vi "SensorSimulationTool.vi"() -> ()   [LabVIEW 2023]
panel:
  in  "ClientUI":enum32{"Page 2"}(tab)
  in  "Bypass1":bool
  in  "Bypass2":bool
  in  "Bypass3":bool
  in  "Bypass4":bool
  in  "Bypass5":bool
  in  "Bypass6":bool
  in  "Tamper1":bool
  in  "Tamper2":bool
  in  "Tamper3":bool
  in  "Tamper4":bool
  in  "Tamper5":bool
  in  "Tamper6":bool
  in  "Alarm1":bool
  in  "Alarm2":bool
  in  "Alarm4":bool
  in  "Alarm5":bool
  in  "Alarm6":bool
  in  "stop":bool
  in  "Alarm3":bool
  # "Zone Sensor Simulation Panel"
  # "1"
  # "2"
  # "3"
  # "4"
  # "5"
  # "6"
  # "Zone"
  # "Alarm Switches"
  # "Bypass Switches"
  # "Tamper Switches"
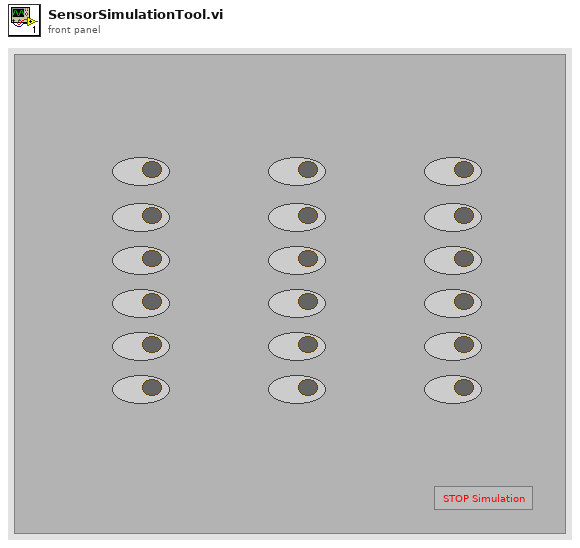
[diagram p1: front panel]
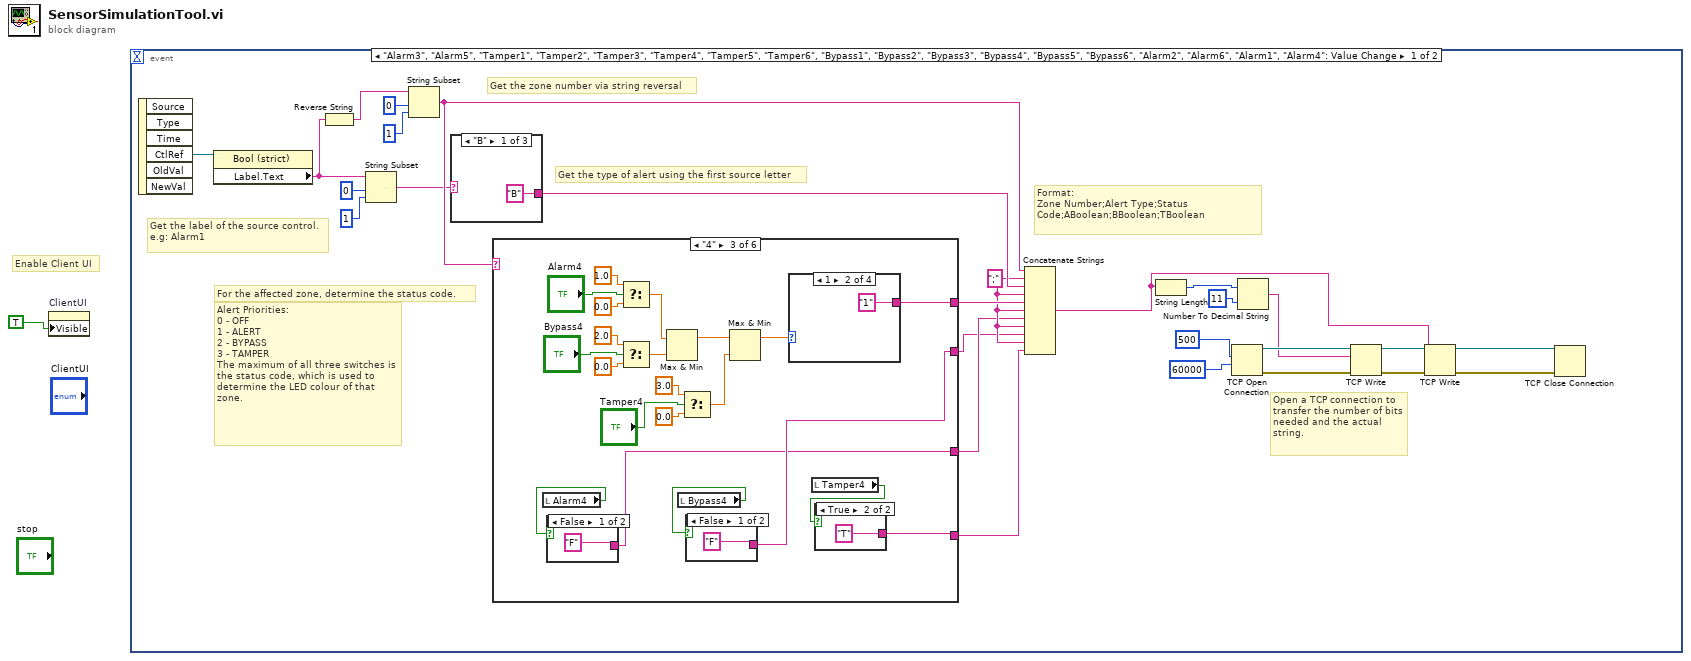
[diagram p0: block diagram]
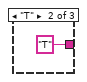
[diagram p2: hidden frame]
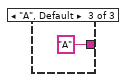
[diagram p3: hidden frame]
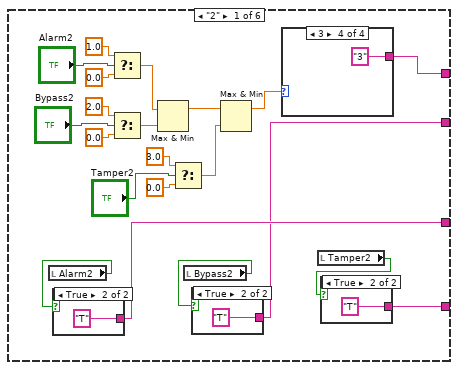
[diagram p4: hidden frame]
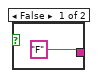
[diagram p5: hidden frame]
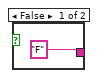
[diagram p6: hidden frame]
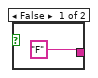
[diagram p7: hidden frame]
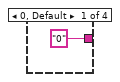
[diagram p8: hidden frame]
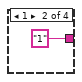
[diagram p9: hidden frame]
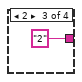
[diagram p10: hidden frame]
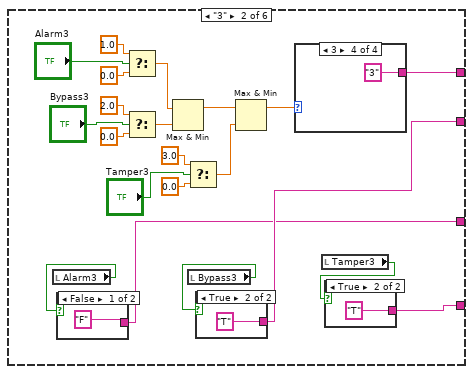
[diagram p11: hidden frame]
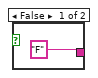
[diagram p12: hidden frame]
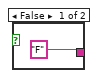
[diagram p13: hidden frame]
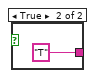
[diagram p14: hidden frame]
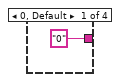
[diagram p15: hidden frame]
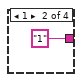
[diagram p16: hidden frame]
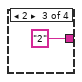
[diagram p17: hidden frame]
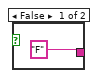
[diagram p18: hidden frame]
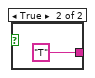
[diagram p19: hidden frame]
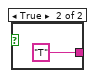
[diagram p20: hidden frame]
diagram:
  # "Enable Client UI"
  n1 = property on="ClientUI" class="TabCtl (strict)"("Visible"=TRUE) -> ()  [unwired: 2 in, 2 out]
  n2 = event shown="[0] \"Alarm3\", \"Alarm5\", \"Tamper1\", \"Tamper2\", \"Tamper3\", \"Tamper4\", \"Tamper5\", \"Tamper6\", \"Bypass1\", \"Bypass2\", \"Bypass3\", \"Bypass4\", \"Bypass5\", \"Bypass6\", \"Alarm2\", \"Alarm6\", \"Alarm1\", \"Alarm4\": Value Change" {
    selector: _ -> [_ _]
    dyn-events: _ -> [_ _]
    timeout: _ -> [_ _]
    event "Alarm3", "Alarm5", "Tamper1", "Tamper2", "Tamper3", "Tamper4", "Tamper5", "Tamper6", "Bypass1", "Bypass2", "Bypass3", "Bypass4", "Bypass5", "Bypass6", "Alarm2", "Alarm6", "Alarm1", "Alarm4": Value Change {
      w8 = ";" ("string")
      # "Open a TCP connection to transfer the number of bits needed and the actual string."
      # "Alert Priorities:\n0 - OFF\n1 - ALERT\n2 - BYPASS\n3 - TAMPER\nThe maximum of all three switches is the status code, which is used to determine the LED colour of that zone."
      # "For the affected zone, determine the status code."
      # "Get the type of alert using the first source letter"
      # "Get the zone number via string reversal"
      # "Get the label of the source control. e.g: Alarm1"
      # "Format:\nZone Number;Alert Type;Status Code;ABoolean;BBoolean;TBoolean"
      n3 = event-data() -> ("CtlRef"=w22:refnum<vi>)  [unwired: 1 in, 5 out]
      n4 = property class="Bool (strict)"(reference=w22) -> ("Label.Text"=w15:string)  [unwired: 1 in, 2 out]
      n5 = Reverse String(1:w15) -> (0:w19:string)
      n6 = String Subset(string=w15, offset (0)=0, length (rest)=1 ("length (rest)")) -> (substring=w12:string)
      n7 = String Subset(string=w19, offset (0)=0, length (rest)=1 ("length (rest)")) -> (substring=w16:string)
      n8 = case shown="\"B\"" w12 {
        tunnel: ["B" ("string") "T" ("string") "A" ("string")] -> w10
        frame "B" {
        }
        frame "T" {
        }
        frame "A", Default {
        }
      }
      n9 = case shown="\"4\"" w16 {
        tunnel: [w41 w72 w100 w134 w162 w193] -> w11
        tunnel: [w33 w63 w94 w125 w156 w187] -> w7
        tunnel: [w32 w64 w95 w126 w157 w188] -> w6
        tunnel: [w37 w68 w99 w130 w161 w192] -> w5
        frame "2" {
          n10 = local read "Alarm2"() -> (w36:bool)
          n11 = case shown="True" w36 {
            tunnel: ["F" "T"] -> w33
            frame False {
            }
            frame True {
            }
          }
          n12 = Select(t=1.0, s="Alarm2", f=0.0) -> (s? t:f=w46:dbl)
          n13 = Select(t=2.0, s="Bypass2", f=0.0) -> (s? t:f=w45:dbl)
          n14 = Max & Min(x=w46, y=w45) -> (max(x,y)=w44:dbl)  [unwired: 1 out]
          n15 = Select(t=3.0, s="Tamper2", f=0.0) -> (s? t:f=w43:dbl)
          n16 = local read "Bypass2"() -> (w35:bool)
          n17 = case shown="True" w35 {
            tunnel: ["F" "T"] -> w32
            frame False {
            }
            frame True {
            }
          }
          n18 = Max & Min(x=w44, y=w43) -> (max(x,y)=w42:dbl)  [unwired: 1 out]
          n19 = case shown="3" w42 {
            tunnel: ["0" "1" "2" "3"] -> w41
            frame 0, Default {
            }
            frame 1 {
            }
            frame 2 {
            }
            frame 3 {
            }
          }
          n20 = local read "Tamper2"() -> (w34:bool)
          n21 = case shown="True" w34 {
            tunnel: ["F" "T"] -> w37
            frame False {
            }
            frame True {
            }
          }
        }
        frame "3" {
          n22 = local read "Alarm3"() -> (w67:bool)
          n23 = case shown="False" w67 {
            tunnel: ["F" "T"] -> w63
            frame False {
            }
            frame True {
            }
          }
          n24 = Select(t=1.0, s="Alarm3", f=0.0) -> (s? t:f=w77:dbl)
          n25 = Select(t=2.0, s="Bypass3", f=0.0) -> (s? t:f=w76:dbl)
          n26 = Max & Min(x=w77, y=w76) -> (max(x,y)=w75:dbl)  [unwired: 1 out]
          n27 = Select(t=3.0, s="Tamper3", f=0.0) -> (s? t:f=w74:dbl)
          n28 = local read "Bypass3"() -> (w66:bool)
          n29 = case shown="True" w66 {
            tunnel: ["F" "T"] -> w64
            frame False {
            }
            frame True {
            }
          }
          n30 = Max & Min(x=w75, y=w74) -> (max(x,y)=w73:dbl)  [unwired: 1 out]
          n31 = case shown="3" w73 {
            tunnel: ["0" "1" "2" "3"] -> w72
            frame 0, Default {
            }
            frame 1 {
            }
            frame 2 {
            }
            frame 3 {
            }
          }
          n32 = local read "Tamper3"() -> (w65:bool)
          n33 = case shown="True" w65 {
            tunnel: ["F" "T"] -> w68
            frame False {
            }
            frame True {
            }
          }
        }
        frame "4" {
          n34 = local read "Alarm4"() -> (w98:bool)
          n35 = case shown="False" w98 {
            tunnel: ["F" "T"] -> w94
            frame False {
            }
            frame True {
            }
          }
          n36 = Select(t=1.0, s="Alarm4", f=0.0) -> (s? t:f=w108:dbl)
          n37 = Select(t=2.0, s="Bypass4", f=0.0) -> (s? t:f=w107:dbl)
          n38 = Max & Min(x=w108, y=w107) -> (max(x,y)=w106:dbl)  [unwired: 1 out]
          n39 = local read "Bypass4"() -> (w97:bool)
          n40 = Select(t=3.0, s="Tamper4", f=0.0) -> (s? t:f=w105:dbl)
          n41 = case shown="False" w97 {
            tunnel: ["F" "T"] -> w95
            frame False {
            }
            frame True {
            }
          }
          n42 = Max & Min(x=w106, y=w105) -> (max(x,y)=w104:dbl)  [unwired: 1 out]
          n43 = case shown="1" w104 {
            tunnel: ["0" "1" "2" "3"] -> w100
            frame 0, Default {
            }
            frame 1 {
            }
            frame 2 {
            }
            frame 3 {
            }
          }
          n44 = local read "Tamper4"() -> (w96:bool)
          n45 = case shown="True" w96 {
            tunnel: ["F" "T"] -> w99
            frame False {
            }
            frame True {
            }
          }
        }
        frame "5" {
          n46 = local read "Alarm5"() -> (w129:bool)
          n47 = case shown="True" w129 {
            tunnel: ["F" "T"] -> w125
            frame False {
            }
            frame True {
            }
          }
          n48 = Select(t=1.0, s="Alarm5", f=0.0) -> (s? t:f=w139:dbl)
          n49 = Select(t=2.0, s="Bypass5", f=0.0) -> (s? t:f=w138:dbl)
          n50 = Max & Min(x=w139, y=w138) -> (max(x,y)=w137:dbl)  [unwired: 1 out]
          n51 = local read "Bypass5"() -> (w128:bool)
          n52 = case shown="False" w128 {
            tunnel: ["F" "T"] -> w126
            frame False {
            }
            frame True {
            }
          }
          n53 = Select(t=3.0, s="Tamper5", f=0.0) -> (s? t:f=w136:dbl)
          n54 = Max & Min(x=w137, y=w136) -> (max(x,y)=w135:dbl)  [unwired: 1 out]
          n55 = case shown="1" w135 {
            tunnel: ["0" "1" "2" "3"] -> w134
            frame 0, Default {
            }
            frame 1 {
            }
            frame 2 {
            }
            frame 3 {
            }
          }
          n56 = local read "Tamper5"() -> (w127:bool)
          n57 = case shown="False" w127 {
            tunnel: ["F" "T"] -> w130
            frame False {
            }
            frame True {
            }
          }
        }
        frame "6" {
          n58 = local read "Alarm6"() -> (w160:bool)
          n59 = case shown="False" w160 {
            tunnel: ["F" "T"] -> w156
            frame False {
            }
            frame True {
            }
          }
          n60 = Select(t=1.0, s="Alarm6", f=0.0) -> (s? t:f=w172:dbl)
          n61 = Select(t=2.0, s="Bypass6", f=0.0) -> (s? t:f=w173:dbl)
          n62 = local read "Bypass6"() -> (w159:bool)
          n63 = Max & Min(x=w172, y=w173) -> (max(x,y)=w174:dbl)  [unwired: 1 out]
          n64 = case shown="True" w159 {
            tunnel: ["F" "T"] -> w157
            frame False {
            }
            frame True {
            }
          }
          n65 = Select(t=3.0, s="Tamper6", f=0.0) -> (s? t:f=w175:dbl)
          n66 = Max & Min(x=w174, y=w175) -> (max(x,y)=w176:dbl)  [unwired: 1 out]
          n67 = case shown="3" w176 {
            tunnel: ["0" "1" "2" "3"] -> w162
            frame 0, Default {
            }
            frame 1 {
            }
            frame 2 {
            }
            frame 3 {
            }
          }
          n68 = local read "Tamper6"() -> (w158:bool)
          n69 = case shown="False" w158 {
            tunnel: ["F" "T"] -> w161
            frame False {
            }
            frame True {
            }
          }
        }
        frame "1", Default {
          # "Get the individual booleans of each switch"
          # "Determine the status code"
          n70 = local read "Alarm1"() -> (w191:bool)
          n71 = case shown="True" w191 {
            tunnel: ["F" "T"] -> w187
            frame False {
            }
            frame True {
            }
          }
          n72 = Select(t=1.0, s="Alarm1", f=0.0) -> (s? t:f=w198:dbl)
          n73 = Select(t=2.0, s="Bypass1", f=0.0) -> (s? t:f=w197:dbl)
          n74 = Max & Min(x=w198, y=w197) -> (max(x,y)=w196:dbl)  [unwired: 1 out]
          n75 = local read "Bypass1"() -> (w190:bool)
          n76 = Select(t=3.0, s="Tamper1", f=0.0) -> (s? t:f=w195:dbl)
          n77 = case shown="False" w190 {
            tunnel: ["F" "T"] -> w188
            frame False {
            }
            frame True {
            }
          }
          n78 = Max & Min(x=w196, y=w195) -> (max(x,y)=w194:dbl)  [unwired: 1 out]
          n79 = case shown="3" w194 {
            tunnel: ["0" "1" "2" "3"] -> w193
            frame 0, Default {
            }
            frame 1 {
            }
            frame 2 {
            }
            frame 3 {
            }
          }
          n80 = local read "Tamper1"() -> (w189:bool)
          n81 = case shown="True" w189 {
            tunnel: ["F" "T"] -> w192
            frame False {
            }
            frame True {
            }
          }
        }
      }
      n82 = Concatenate Strings "Concatenate Strings"(w16, w8, w10, w8, w11, w8, w7, w8, w6, w8, w5) -> (w4:string)
      n83 = String Length(string=w4) -> (length=w9:i32)
      n84 = TCP Open Connection(remote port or service name=u16 500, timeout ms (60000)=60000) -> (connection ID=w26:refnum<k5>, error out=w25:errorcluster)  [unwired: 3 in]
      n85 = Number To Decimal String(number=w9, width (-)=i16 11) -> (decimal integer string=w21:string)
      n86 = TCP Write(connection ID=w26, data in=w21, error in (no error)=w25) -> (connection ID out=w23:refnum<k5>, error out=w24:errorcluster)  [unwired: 1 in, 1 out]
      n87 = TCP Write(connection ID=w23, data in=w4, error in (no error)=w24) -> (connection ID out=w2:refnum<k5>, error out=w3:errorcluster)  [unwired: 1 in, 1 out]
      n88 = TCP Close Connection(connection ID=w2, error in (no error)=w3) -> ()  [unwired: 1 in, 2 out]
    }
    event "stop": Mouse Up {
      # "Stop simulation"
      n89 = event-data() -> ()  [unwired: 1 in, 8 out]
      n90 = Stop() -> ()  [unwired: 1 in]
    }
  }
